vi "graph.vi"() -> ()   [LabVIEW 2018]
panel:
  out "Graph":i32[](graph)
  out "testVal":i32=3
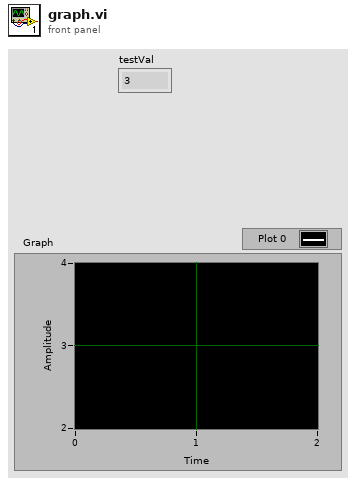
[diagram p1: front panel]
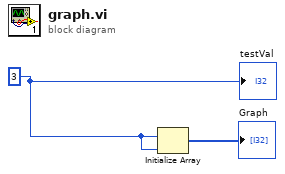
[diagram p0: block diagram]
diagram:
  w2 = 3
  n1 = Initialize Array(w2, w2) -> (→"Graph":i32[])
  "testVal" <- w2
